vi "Setting.vi"(6 "Website":string, 7 "Product_Ref":string, 8 "error in (no error)":errorcluster, 9 "Secret Key for License Verification Requests":string, 10 "Secret Key for License Creation":string, 11 "Abstract License in":refnum<class "Software License Manager.lvclass">) -> (0 "error out":errorcluster, 3 "Abstract License out":refnum<class "Software License Manager.lvclass">)   [LabVIEW 2021, in "Software License Manager.lvclass"]
uses:
  Software License Manager.lvclass
  Software License Manager.lvclass/Software License Manager.ctl
  Board/Board.lvclass
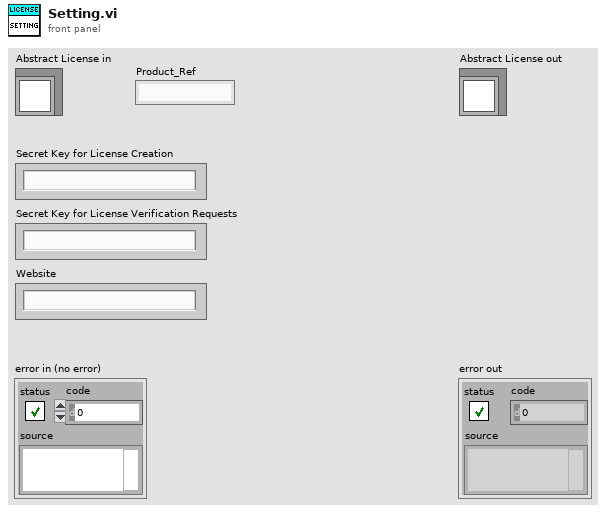
[diagram p1: front panel]
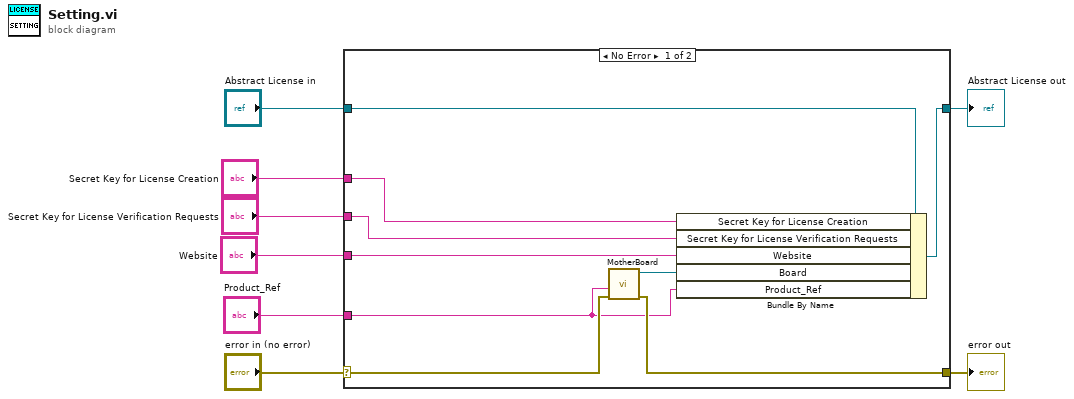
[diagram p0: block diagram]
diagram:
  n1 = case shown="No Error" "error in (no error)" {
    selector: "error in (no error)" -> [w15 w19]
    tunnel: [w14 w19] -> w7
    tunnel: [w16 w18] -> w5
    tunnel: "Abstract License in" -> [w11 w18]
    tunnel: "Website" -> [w17 _]
    tunnel: "Secret Key for License Verification Requests" -> [w10 _]
    tunnel: "Secret Key for License Creation" -> [w9 _]
    tunnel: "Product_Ref" -> [w12 _]
    frame No Error {
      n2 = call "MotherBoard.vi"("error in (no error)"=w15, "Product_Ref"=w12) -> ("error out"=w14:errorcluster, "Board out"=w13:refnum<class "Board.lvclass">)  [unwired: 8 in]
      n3 = Bundle By Name(cluster=w11, "Secret Key for License Creation"=w9, "Secret Key for License Verification Requests"=w10, "Website"=w17, "Board"=w13, "Product_Ref"=w12) -> (w16:refnum<class "Software License Manager.lvclass">)
    }
    frame Error {
    }
  }
  "error out" <- w7
  "Abstract License out" <- w5
